vi "Pulse Mode - Read Range.vi"(8 "error in (no error)":errorcluster, 11 "VISA resource name":refnum<visa-resource-name>) -> (0 "error out":errorcluster, 2 "Trigger Source":u16(ring) items=["AUTO", "HIGH", "LOW"], 3 "VISA resource name out":refnum<visa-resource-name>)   [LabVIEW 2014, in "Associated Power Technologies 8500 Series.lvlib"]
doc: "Get the range configuration of pulse mode."
uses:
  <instrlib>/Associated Power Technologies 8500 Series/Associated Power Technologies 8500 Series.lvlib
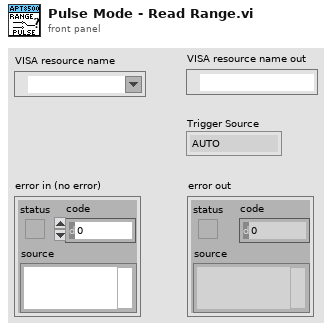
[diagram p1: front panel]
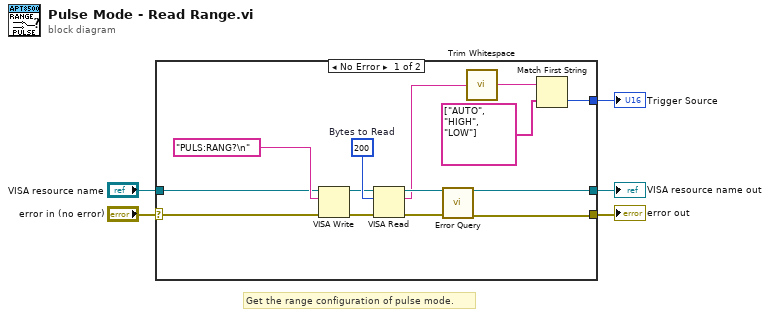
[diagram p0: block diagram]
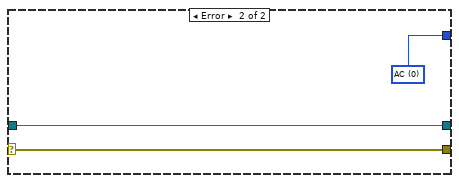
[diagram p2: hidden frame]
diagram:
  # "Get the range configuration of pulse mode."
  n1 = case shown="No Error" "error in (no error)" {
    selector: "error in (no error)" -> [w15 w22]
    tunnel: [w10 w22] -> w3
    tunnel: [w13 w21] -> w2
    tunnel: "VISA resource name" -> [w14 w21]
    tunnel: [w7 w20] -> w1
    frame No Error {
      w19 = u32 200  # Bytes to Read
      n2 = VISA Write(VISA resource name=w14, write buffer="PULS:RANG?\n", error in (no error)=w15) -> (VISA resource name out=w17:refnum<visa-resource-name>, error out=w18:errorcluster)  [unwired: 1 out]
      n3 = VISA Read(VISA resource name=w17, byte count=w19, error in (no error)=w18) -> (VISA resource name out=w12:refnum<visa-resource-name>, read buffer=w9:string, error out=w11:errorcluster)  [unwired: 1 out]
      n4 = call <instrlib>:"Error Query.vi"("VISA resource name"=w12, "error in (no error)"=w11) -> ("VISA resource name out"=w13:refnum<visa-resource-name>, "error out"=w10:errorcluster)  [unwired: 10 in, 2 out]
      n5 = call <vilib>:"Trim Whitespace.vi"("string"=w9) -> ("trimmed string"=w8:string)  [unwired: 1 in]
      n6 = Match First String(2:string[] ["AUTO", "HIGH", "LOW"] ("string array"), 3:w8) -> (0:w7:i32)  [unwired: 1 out]
    }
    frame Error {
      w20 = u16 0 items=["AC", "DC", "ACDC"] ("Couple")
    }
  }
  "VISA resource name out" <- w2
  "error out" <- w3
  "Trigger Source" <- w1
